vi "WPI_DriverStationGet Alliance Info.vi"() -> (0 "Match Type":T1, 1 "Match Number":u16, 2 "Position":T2, 3 "Alliance":T3, 4 "Replay Number":u16, 5 "Event Name":string)   [LabVIEW 2017]
doc: "Returns the team alliance and field position of the robot. Also returns match information.\n\nThis software is licensed. Open the labview\\readme\\WPI Robotics Library Open Source License.txt file for more information."
uses:
  <vilib>/Rock Robotics/WPI/DriverStation/WPI_DriverStationAllianceInfo.ctl
  <vilib>/Rock Robotics/WPI/DriverStation/WPI_DriverStationPositionInfo.ctl
  <vilib>/Rock Robotics/SystemInterfaces/NetworkCommunication/NetComm_MatchType.ctl
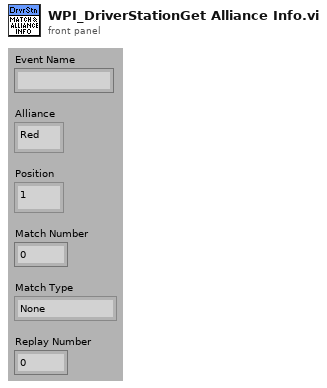
[diagram p1: front panel]
types:
  T1 = typedef "NetComm_MatchType.ctl" = enum32{"None", "Practice", "Qualification", "Elimination"}
  T2 = typedef "WPI_DriverStationPositionInfo.ctl" = enum16{"1", "2", "3"}
  T3 = typedef "WPI_DriverStationAllianceInfo.ctl" = enum16{"Red", "Blue", "Invalid"}
  T4 = typedef "NetComm_AllianceStation.ctl" = enum16{"Red 1", "Red 2", "Red 3", "Blue 1", "Blue 2", "Blue 3"}
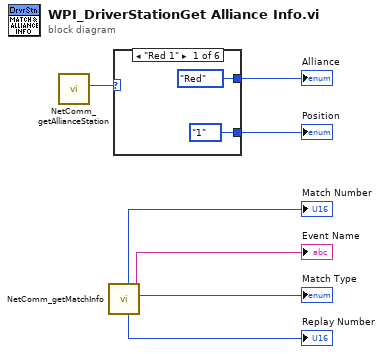
[diagram p0: block diagram]
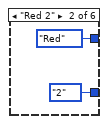
[diagram p2: hidden frame]
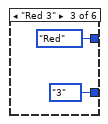
[diagram p3: hidden frame]
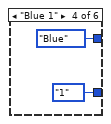
[diagram p4: hidden frame]
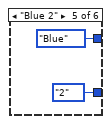
[diagram p5: hidden frame]
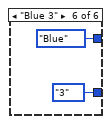
[diagram p6: hidden frame]
diagram:
  n1 = call <vilib>:"NetComm_getAllianceStation.vi"() -> ("Alliance Station"=w7:T4)  [unwired: 10 in, 1 out]
  n2 = call <vilib>:"NetComm_getMatchInfo.vi"() -> ("Match Type"=→"Match Type":T1, "Event Name"=→"Event Name":string, "Replay Number"=→"Replay Number":u16, "Match Number"=→"Match Number":u16)  [unwired: 6 in, 2 out]
  n3 = case shown="\"Red 1\"" w7 {
    tunnel: [WPI_DriverStationAllianceInfo."Red" ("Alliance") WPI_DriverStationAllianceInfo."Red" ("Alliance") WPI_DriverStationAllianceInfo."Red" ("Alliance") WPI_DriverStationAllianceInfo."Blue" ("Alliance") WPI_DriverStationAllianceInfo."Blue" ("Alliance") WPI_DriverStationAllianceInfo."Blue" ("Alliance")] -> w6
    tunnel: [WPI_DriverStationPositionInfo."1" ("Position") WPI_DriverStationPositionInfo."2" ("Position") WPI_DriverStationPositionInfo."3" ("Position") WPI_DriverStationPositionInfo."1" ("Position") WPI_DriverStationPositionInfo."2" ("Position") WPI_DriverStationPositionInfo."3" ("Position")] -> w5
    frame "Red 1" {
    }
    frame "Red 2" {
    }
    frame "Red 3" {
    }
    frame "Blue 1" {
    }
    frame "Blue 2" {
    }
    frame "Blue 3" {
    }
  }
  "Alliance" <- w6
  "Position" <- w5
